vi "Stop UUDT Engine.vi"(11 "vi reference":refnum<vi>) -> ()   [LabVIEW 2024, in "GMLAN.lvlib"]
uses:
  GMLAN.lvlib
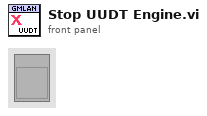
[diagram p1: front panel]
types:
  T1 = enum32{"Bad", "Idle", "Run top level", "Running"}
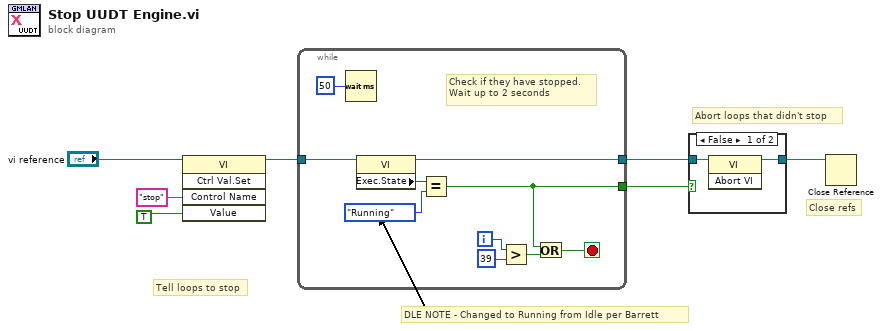
[diagram p0: block diagram]
diagram:
  # "Close refs"
  # "Abort loops that didn't stop"
  # "DLE NOTE - Changed to Running from Idle per Barrett"
  # "Tell loops to stop"
  n1 = invoke class="VI" method="Ctrl Val.Set"(reference="vi reference", "Control Name"="stop", "Value"=TRUE ("force destroy? (F)")) -> (reference out=w6:refnum<vi>)  [unwired: 2 in, 4 out]
  n2 = while {
    tunnel: w6 -> [w16]
    tunnel: [w15] -> w4
    tunnel: [w8] -> w5
    i -> [w13]
    stop <- w14 stop-if-true
    # "Check if they have stopped.\nWait up to 2 seconds"
    n3 = Wait (ms)(milliseconds to wait=u32 50) -> ()  [unwired: 1 out]
    n4 = property class="VI"(reference=w16) -> (reference out=w15:refnum<vi>, "Exec.State"=w10:T1)  [unwired: 1 in, 1 out]
    n5 = Equal?(x=w10, y=T1."Running") -> (x = y?=w8:bool)
    n6 = Greater?(x=w13, y=39) -> (0:w11:bool)
    n7 = Or(x=w8, y=w11) -> (x .or. y?=w14:bool)
  }
  n8 = case shown="False" w5 {
    tunnel: w4 -> [w19 w20]
    tunnel: [w18 w20] -> w1
    frame False {
      n9 = invoke class="VI" method="Abort VI"(reference=w19) -> (reference out=w18:refnum<vi>)  [unwired: 2 in, 2 out]
    }
    frame True {
    }
  }
  n10 = Close Reference(reference=w1) -> ()  [unwired: 1 in, 1 out]
